vi "Get settings chain.vi"(8 "error in (no error)":errorcluster, 11 "TemplateBase in":refnum<class "Template.lvclass">) -> (0 "error out":errorcluster, 1 "class name":string[](array[string]), 2 "settings":variant[](array[variant]), 3 "TemplateBase out":refnum<class "Template.lvclass">)   [LabVIEW 2012, in "Template.lvclass"]
doc: "Returns an array of variants containing the settings clusters of each class in the inheritance chain (lowest child class first), together with an array of all class names in the inheritance chain.\n\nFor classes without settings cluster, the settings chain contains empty variants."
uses:
  Template.lvclass
  <vilib>/Distrio/Murmex/Murmex/Murmex.lvclass
  Template.lvclass/Template.ctl
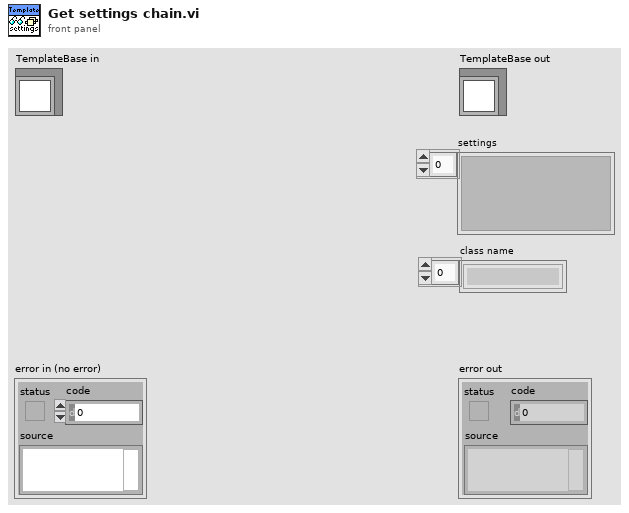
[diagram p1: front panel]
types:
  T1 = typedef "Template.lvclass/settings_cluster.ctl" = cluster{"parameter":string}
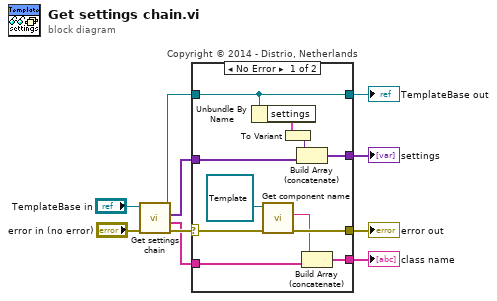
[diagram p0: block diagram]
diagram:
  n1 = call-parent "Get settings chain.vi"("error in (no error)"="error in (no error)", "MurmexBase in"="TemplateBase in") -> ("error out"=w8:errorcluster, "class name"=w5:string[], "settings"=w6:variant[], "MurmexBase out"=w7:refnum<class "Template.lvclass">)  [unwired: 6 in]
  n2 = case "Copyright © 2014 - Distrio, Netherlands" shown="No Error" w8 {
    selector: w8 -> [w21 w23]
    tunnel: [w20 w23] -> w3
    tunnel: [w14 w22] -> w4
    tunnel: w7 -> [w14 w22]
    tunnel: [w18 _] -> w1
    tunnel: [w17 _] -> w2
    tunnel: w6 -> [w15 _]
    tunnel: w5 -> [w16 _]
    frame No Error {
      n3 = Unbundle By Name(w14) -> ("settings"=w13:T1)
      n4 = call <vilib>:"Get component name.vi"("error in (no error)"=w21, "Murmex in"=refnum<class "Template.lvclass"> refnum ("TemplateBase out")) -> ("error out"=w20:errorcluster, "component name"=w19:string)  [unwired: 7 in, 1 out]
      n5 = To Variant(anything=w13) -> (Variant=w12:variant)
      n6 = Build Array (concatenate)(w12, w15) -> (w17:variant[])
      n7 = Build Array (concatenate)(w19, w16) -> (w18:string[])
    }
    frame Error {
    }
  }
  "error out" <- w3
  "TemplateBase out" <- w4
  "settings" <- w2
  "class name" <- w1
